vi "SEK2019v1Reto.vi"(10 "NXT/EV3":T1, 11 "PortGyro":T2 items=["Port 1", "Port 2", "Port 3", "Port 4"]) -> (2 "NXT/EV3 2":T1)   [LabVIEW 2016]
uses:
  <vilib>/NXT/Subs/LVHSConnector.ctl
  <vilib>/NXT/LegoClasses/BrickReference/BrickReference.lvclass
  <vilib>/NXT/Block Support/NXT_InputPort.ctl
  <vilib>/NXT/Block Support/NXT_OutputPort.ctl
  <vilib>/NXT/Dual Mode Library/Sensors/EV3_Gyro_Angle.vi
  <vilib>/NXT/NXTIO Xnodes/NXTIONodeSubVIs/NXTMoveMotors.vi
  <vilib>/NXT/NXTIO Xnodes/AddressXNode/NXTIOAddress.xnode
  <vilib>/NXT/NXTIO Xnodes/NXTIOXNode/NXTIO.xnode
panel:
  in  "inicial":sgl
  in  "Kd":sgl
  in  "Ki":sgl
  in  "Kp":sgl=2.0
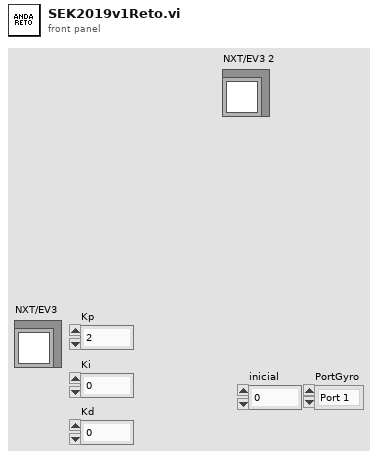
[diagram p1: front panel]
types:
  T1 = typedef "LVHSConnector.ctl" = refnum<class "BrickReference.lvclass">
  T2 = typedef "NXT_InputPort.ctl" = u32
  T3 = typedef "NXT_OutputPort.ctl" = u8
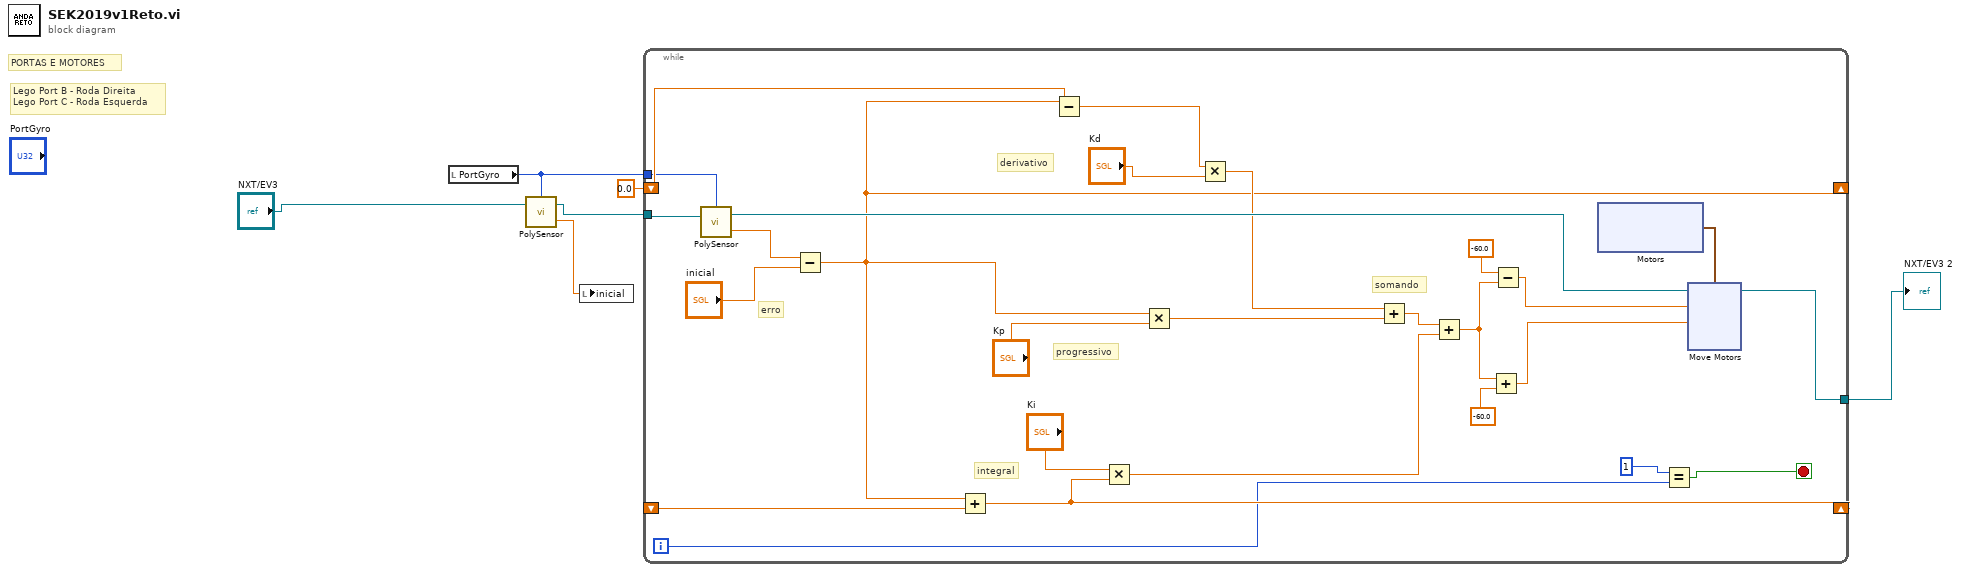
[diagram p0: block diagram]
diagram:
  # "Lego Port B - Roda Direita\nLego Port C - Roda Esquerda"
  # "PORTAS E MOTORES"
  n1 = local read "PortGyro"() -> (w3:T2)
  n2 = call-poly <vilib>:"PolySensor.vi"("NXT/EV3"="NXT/EV3", "Port (Port 1)"=w3) -> ("Degrees"=w5:sgl, "NXT/EV3"=w6:T1)  [unwired: 1 in]
  n3 = local write "inicial"(w5) -> ()
  n4 = while {
    tunnel: w6 -> [w33]
    shift-right: [w20] -> _
    shift-left: _ -> [w22]
    shift-right: [w14] -> _
    shift-left: sgl 0.0 -> [w17]
    tunnel: w3 -> [w11]
    tunnel: [w10] -> w1
    i -> [w9]
    stop <- w8 stop-if-true
    # "somando"
    # "erro"
    # "progressivo"
    # "integral"
    # "derivativo"
    n5 = call-poly <vilib>:"PolySensor.vi"("NXT/EV3"=w33, "Port (Port 1)"=w11) -> ("Degrees"=w16:sgl, "NXT/EV3"=w23:T1)  [unwired: 1 in]
    n6 = Subtract(x=w16, y="inicial") -> (x-y=w14:sgl)
    n7 = Add(x=w14, y=w22) -> (x+y=w20:sgl)
    n8 = Subtract(x=w14, y=w17) -> (x-y=w12:sgl)
    n9 = Multiply(x="Ki", y=w20) -> (x*y=w19:sgl)
    n10 = Multiply(x=w14, y="Kp") -> (x*y=w26:sgl)
    n11 = Multiply(x=w12, y="Kd") -> (x*y=w18:sgl)
    n12 = Add(x=w18, y=w26) -> (x+y=w24:sgl)
    n13 = Add(x=w24, y=w19) -> (x+y=w25:sgl)
    n14 = Add(x=w25, y=sgl -60.0) -> (x+y=w27:sgl)
    n15 = Subtract(x=sgl -60.0, y=w25) -> (x-y=w30:sgl)
    n16 = xnode "Motors"() -> ("Motor"=w32:cluster{"Port":T3, "Port":T3})
    n17 = Equal?(x=1, y=w9) -> (x = y?=w8:bool)
    n18 = xnode "Move Motors"("Power/Speed 2"=w27, "Power/Speed 1"=w30, "Motors"=w32, "NXT/EV3"=w23) -> ("NXT/EV3"=w10:T1)
  }
  "NXT/EV3 2" <- w1
